vi "Return Term Settings.vi"(8 "error in (no error)":errorcluster {"code" format="Error %.0f"}, 10 "Term":string, 11 "Printer in":refnum<class "VIDoc Printer.lvclass">) -> (0 "error out":errorcluster {"code" format="Error %.0f"}, 1 "Found?":bool, 2 "Term Settings":T1={"Memory"=TRUE, "By Folder"=TRUE, "By Tree"=TRUE, "By List"=TRUE, "Methods"=TRUE, "Method Options"={"Front Panels"=TRUE, "Options"=TRUE, "Controls"=TRUE}, "List Detail Level"=enum."None", "Methods Detail Level"=enum."None", "Controls Detail Level"=enum."None"}, 3 "Printer out":refnum<class "VIDoc Printer.lvclass">)   [LabVIEW 2023, in "VIDoc Printer.lvlib" / "VIDoc Printer.lvclass"]
uses:
  VIDoc Printer.lvclass
  Settings/Printer Settings/Detail Level Enum.ctl
  Settings/Printer Settings/Printer Settings.lvclass
  Settings/Printer Settings/VI Settings.ctl
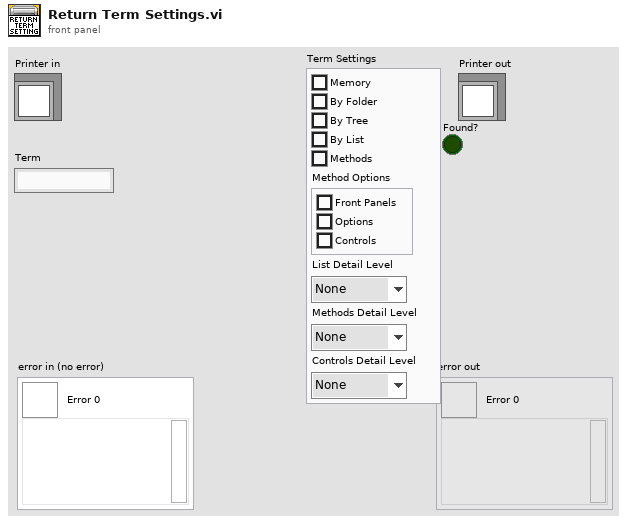
[diagram p1: front panel]
types:
  T1 = typedef "VIDoc Printer.lvlib/Printer Settings.lvclass/VI Settings.ctl" = cluster{"Memory":bool, "By Folder":bool, "By Tree":bool, "By List":bool, "Methods":bool, "Method Options":cluster{"Front Panels":bool, "Options":bool, "Controls":bool}, "List Detail Level":T2, "Methods Detail Level":T2, "Controls Detail Level":T2}
  T2 = typedef "VIDoc Printer.lvlib/Printer Settings.lvclass/Detail Level Enum.ctl" = enum16{"None", "Minimal", "Standard", "Full"}
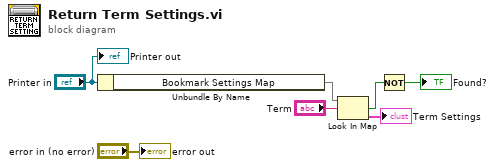
[diagram p0: block diagram]
diagram:
  n1 = Unbundle By Name("Printer in") -> ("Bookmark Settings Map"=w4:map{string, T1})
  n2 = Look In Map(map=w4, key="Term") -> (key not found?=w2:bool, value=→"Term Settings":T1)  [unwired: 1 in]
  n3 = Not(x=w2) -> (.not. x?=→"Found?":bool)
  "error out" <- "error in (no error)"
  "Printer out" <- "Printer in"
